vi "Configure Hardware.vi"(8 "error in":errorcluster, 9 "Sleep Capability":u32(ring) items=["Disabled", "Enabled"], 10 "Link Speed":u32(ring)=1 items=["100Mb/s"=1, "1000Mb/s"=2], 11 "XNET Interface":refnum<k21>="ENET1") -> (0 "error out":errorcluster, 2 "Sleep Capability Configured":u32(ring) items=["Disabled", "Enabled"], 3 "Link Speed Configured":u32(ring)=1 items=["100Mb/s"=1, "1000Mb/s"=2])   [LabVIEW 2026]
uses:
  <vilib>/nisyscfg/Save Changes (Hardware).vi
  <vilib>/nisyscfg/Close (Resources).vi
  <vilib>/nisyscfg/Close (Filter).vi
  <vilib>/nisyscfg/Close (System).vi
  <vilib>/nisyscfg/nisyscfg.lvlib
  <resource>/objmgr/niflexrioatomicsae.rc
panel:
  out "Interrupt Moderation":u32(ring) items=["Off", "Low", "Medium", "High"]
  out "Jumbo Frames":u32(ring) items=["Disabled", "9018_bytes"]
  out "Port Mode":u32(ring) items=["Direct", "Tap"]
  out "PHY State":u32(ring) items=["Slave", "Master"]
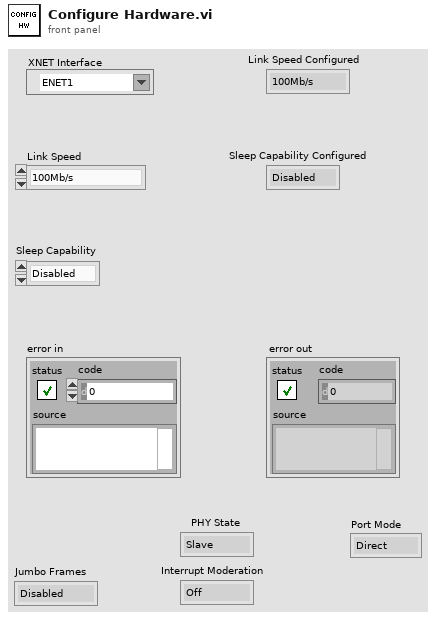
[diagram p1: front panel]
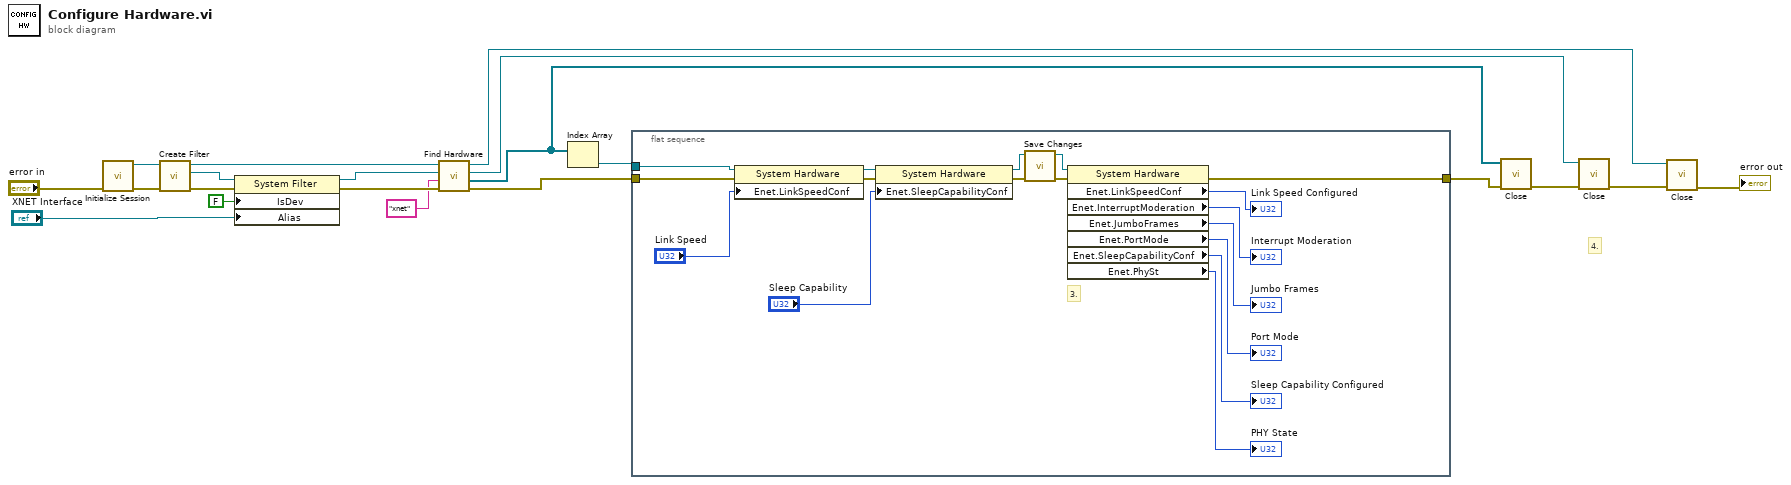
[diagram p0: block diagram]
diagram:
  # "4."
  n1 = call <vilib>:"Initialize Session.vi"("error in (no error)"="error in") -> ("error out"=w18:errorcluster, "Session out"=w17:refnum<k21>)  [unwired: 9 in]
  n2 = call <vilib>:"Create Filter.vi"("error in (no error)"=w18, "Session in"=w17) -> ("error out"=w20:errorcluster, "Filter out"=w19:refnum<k20>, "Session out"=w7:refnum<k21>)  [unwired: 7 in]
  n3 = property class="System Filter"(reference=w19, error in=w20, "IsDev"=FALSE ("Is Device"), "Alias"="XNET Interface") -> (reference out=w14:refnum<k20>, error out=w15:errorcluster)
  n4 = call <vilib>:"Find Hardware.vi"("error in (no error)"=w15, "Experts"="xnet", "Filter in"=w14, "Session in"=w7) -> ("error out"=w11:errorcluster, "Resources out"=w8:refnum<k20>[], "Filter out"=w3:refnum<k20>, "Session out"=w4:refnum<k21>)  [unwired: 4 in]
  n5 = Index Array(array=w8) -> (element=w12:refnum<k20>)  [unwired: 1 in]
  n6 = flat-sequence {
    tunnel: w12 -> [w37]
    tunnel: w11 -> [w36]
    tunnel: [w35] -> w6
    frame #0 {
      # "3."
      n7 = property class="System Hardware"(reference=w37, error in=w36, "Enet.LinkSpeedConf"="Link Speed") -> (reference out=w26:refnum<k20>, error out=w23:errorcluster)
      n8 = property class="System Hardware"(reference=w26, error in=w23, "Enet.SleepCapabilityConf"="Sleep Capability") -> (reference out=w25:refnum<k20>, error out=w22:errorcluster)
      n9 = call-poly <vilib>:"Save Changes.vi"("error in (no error)"=w22, "Resource in"=w25) -> ("error out"=w21:errorcluster, "Resource out"=w24:refnum<k20>)  [unwired: 6 in, 2 out]
      n10 = property class="System Hardware"(reference=w24, error in=w21) -> (error out=w35:errorcluster, "Enet.LinkSpeedConf"=→"Link Speed Configured":u32, "Enet.InterruptModeration"=→"Interrupt Moderation":u32, "Enet.JumboFrames"=→"Jumbo Frames":u32, "Enet.PortMode"=→"Port Mode":u32, "Enet.SleepCapabilityConf"=→"Sleep Capability Configured":u32, "Enet.PhySt"=→"PHY State":u32)  [unwired: 1 out]
    }
  }
  n11 = call-poly <vilib>:"Close.vi"("error in (no error)"=w6, "Resources in"=w8) -> ("error out"=w9:errorcluster)  [unwired: 9 in]
  n12 = call-poly <vilib>:"Close.vi"("error in (no error)"=w9, "Filter in"=w3) -> ("error out"=w5:errorcluster)  [unwired: 9 in]
  n13 = call-poly <vilib>:"Close.vi"("error in (no error)"=w5, "Session in"=w4) -> ("error out"=→"error out":errorcluster)  [unwired: 9 in]
